vi "FMA1600A Get Bank Total Flow.vi"(0 "Integral Array Input 1":dbl[](array[numeric]), 5 "Integral Array Input 2":dbl[](array[numeric]), 7 "Integral Array Input -3":dbl[](array[numeric]), 9 "Min to Sec Convert (Total Flow)":dbl=60.0 format="%#_13g", 11 "error in (no error)":errorcluster, 12 "LPM (Vol. Flow) 1":dbl, 13 "LPM (Vol. Flow) 2":dbl, 14 "LPM (Vol. Flow) 3":dbl) -> (1 "Tot.Flow (Liters) Bank 1":dbl, 2 "Tot.Flow (Liters) Bank 2":dbl, 3 "Tot.Flow (Liters) Bank 3":dbl, 4 "Integral Array Output 1":dbl[](array[numeric]), 6 "Integral Array Output 2":dbl[](array[numeric]), 8 "Integral Array Output-3":dbl[](array[numeric]), 15 "error out":errorcluster)   [LabVIEW 2020]
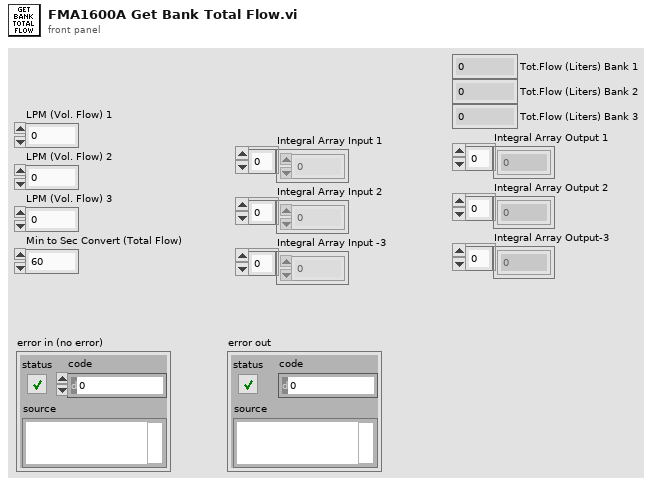
[diagram p1: front panel]
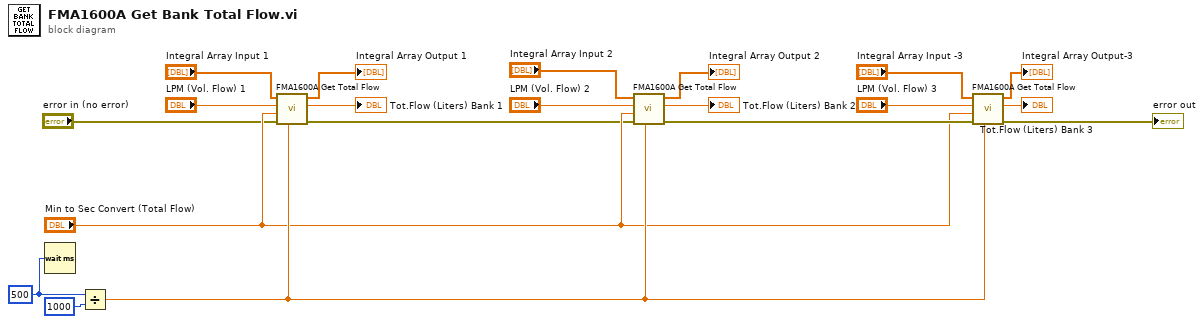
[diagram p0: block diagram]
diagram:
  w4 = u32 500 ("milliseconds to wait")
  n1 = Wait (ms)(milliseconds to wait=w4) -> ()  [unwired: 1 out]
  n2 = Divide(x=w4, y=u32 1000) -> (x/y=w17:dbl)
  n3 = call "FMA1600A Get Total Flow.vi"("Timer"=w17, "error in (no error)"="error in (no error)", "Min to Sec Convert (Total Flow)"="Min to Sec Convert (Total Flow)", "LPM (Vol. Flow)"="LPM (Vol. Flow) 1", "Integral Array Input"="Integral Array Input 1") -> ("error out"=w12:errorcluster, "Integral"=→"Tot.Flow (Liters) Bank 1":dbl, "Integral Array Output"=→"Integral Array Output 1":dbl[])  [unwired: 4 in]
  n4 = call "FMA1600A Get Total Flow.vi"("Timer"=w17, "error in (no error)"=w12, "Min to Sec Convert (Total Flow)"="Min to Sec Convert (Total Flow)", "LPM (Vol. Flow)"="LPM (Vol. Flow) 2", "Integral Array Input"="Integral Array Input 2") -> ("error out"=w16:errorcluster, "Integral"=→"Tot.Flow (Liters) Bank 2":dbl, "Integral Array Output"=→"Integral Array Output 2":dbl[])  [unwired: 4 in]
  n5 = call "FMA1600A Get Total Flow.vi"("Timer"=w17, "error in (no error)"=w16, "Min to Sec Convert (Total Flow)"="Min to Sec Convert (Total Flow)", "LPM (Vol. Flow)"="LPM (Vol. Flow) 3", "Integral Array Input"="Integral Array Input -3") -> ("error out"=→"error out":errorcluster, "Integral"=→"Tot.Flow (Liters) Bank 3":dbl, "Integral Array Output"=→"Integral Array Output-3":dbl[])  [unwired: 4 in]
